vi "get_text_message_value.vi"(8 "error in":errorcluster, 11 "abstract_message_base.lvclass":refnum<class "abstract_message_base.lvclass">) -> (0 "error out":errorcluster, 2 "content":string[](array[string]), 3 "role":string)   [LabVIEW 2020, in "message_text.lvclass"]
uses:
  message_text.lvclass
  abstract_message_base/abstract_message_base.lvclass
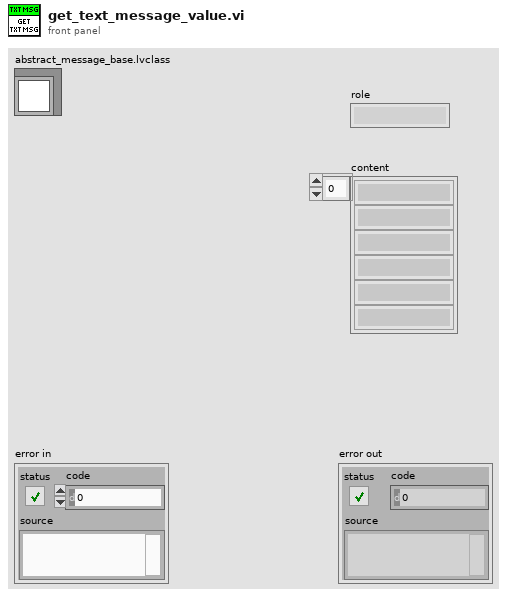
[diagram p1: front panel]
types:
  T1 = typedef "message_text.lvclass/message.ctl" = cluster{"role":string, "content":string[]}
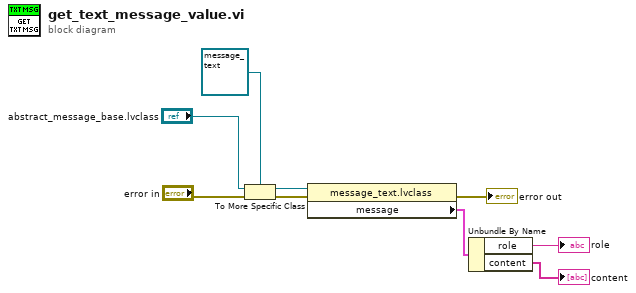
[diagram p0: block diagram]
diagram:
  n1 = To More Specific Class(target class=refnum<class "message_text.lvclass"> refnum ("message_text.lvclass"), reference="abstract_message_base.lvclass", error in="error in") -> (specific class reference=w5:refnum<class "message_text.lvclass">, error out=w6:errorcluster)
  n2 = property class="message_text.lvclass"(reference=w5, error in=w6) -> (error out=→"error out":errorcluster, "message"=w3:T1)  [unwired: 1 out]
  n3 = Unbundle By Name(w3) -> ("role"=→"role":string, "content"=→"content":string[])
